vi "Init.vi"(8 "error in":errorcluster, 11 "NEO480 in":refnum<class "Virtual NEO480.lvclass">) -> (0 "error out":errorcluster, 3 "NEO480 out":refnum<class "Virtual NEO480.lvclass">)   [LabVIEW 2024, in "Virtual NEO480.lvclass"]
uses:
  Virtual NEO480.lvclass
  Virtual NEO480.lvclass/Virtual NEO480.ctl
  Source/Interfaces/IConfiguration/IConfiguration.lvclass
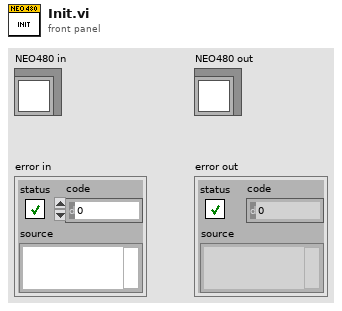
[diagram p1: front panel]
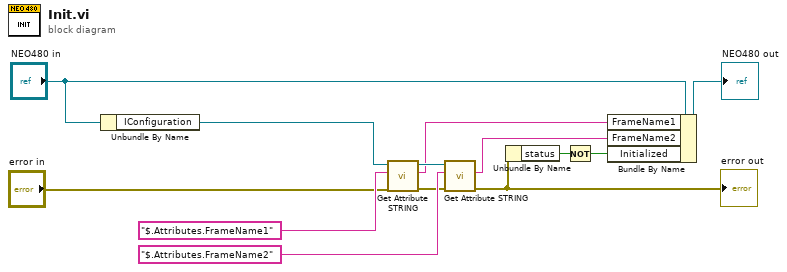
[diagram p0: block diagram]
diagram:
  n1 = Unbundle By Name("NEO480 in") -> ("IConfiguration"=w13:refnum<class "IConfiguration.lvclass">)
  n2 = call-dynamic "Get Attribute STRING.vi"("error in"="error in", "Attribute"="$.Attributes.FrameName1", "IConfiguration in"=w13) -> ("error out"=w7:errorcluster, "Value"=w6:string, "IConfiguration out"=w10:refnum<class "IConfiguration.lvclass">)  [unwired: 6 in]
  n3 = call-dynamic "Get Attribute STRING.vi"("error in"=w7, "Attribute"="$.Attributes.FrameName2", "IConfiguration in"=w10) -> ("error out"=w3:errorcluster, "Value"=w5:string)  [unwired: 6 in, 1 out]
  "error out" <- w3
  n4 = Unbundle By Name(w3) -> ("status"=w2:bool)
  n5 = Not(x=w2) -> (.not. x?=w1:bool)
  n6 = Bundle By Name(cluster="NEO480 in", "FrameName1"=w6, "FrameName2"=w5, "Initialized"=w1) -> (→"NEO480 out":refnum<class "Virtual NEO480.lvclass">)
